vi "Get DI Camera Info.vi"(11 "info":u32) -> (2 "function return":u32, 3 "info out":u32)   [LabVIEW 2018, in "AndorSDK.lvlib"]
doc: "EXPNETTYPE unsigned int WINAPI GetDICameraInfo(void * info);"
uses:
  AndorSDK.lvlib
  ATMCD32D.dll
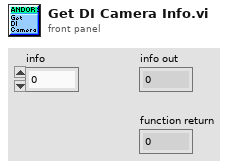
[diagram p1: front panel]
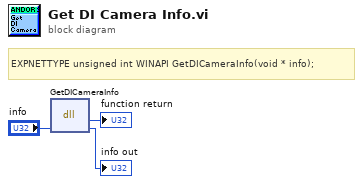
[diagram p0: block diagram]
diagram:
  # "EXPNETTYPE unsigned int WINAPI GetDICameraInfo(void * info);"
  n1 = dll-call lib="PTH2babs E\nPersönliches02 - Arbeit03-HiwijobsLabviewCodelibANDOR\tAndor SDK\nATMCD32D.*" fn="GetDICameraInfo"("info"="info") -> (→"function return":u32, "info"=→"info out":u32)  [unwired: 3 in, 2 out]
